vi "Logger.vi"(0 "Folder":path, 5 "Name":string, 7 "Level":T1=enum."Info", 9 "Retain (days)":i32=14, 11 "Length":i32=10000) -> ()   [LabVIEW 2020]
uses:
  Typedefs/Logger-Level.ctl
  Typedefs/Logger-Queue Data.ctl
  Typedefs/Logger-Action.ctl
  Typedefs/Logger-State.ctl
  Typedefs/Logger-Globals.vi
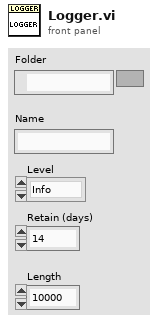
[diagram p1: front panel]
types:
  T1 = typedef "Logger-Level.ctl" = enum16{"Debug", "TCP", "Info", "Warning", "Error", "Critical"}
  T2 = typedef "Logger-Queue Data.ctl" = cluster{"Action":T3, "Level":T1, "Time":dbl, "Message":string}
  T3 = typedef "Logger-Action.ctl" = enum16{"None", "Init", "Add", "Show", "Offset", "Quit"}
  T4 = typedef "Logger-State.ctl" = cluster{"path":path, "index":i32, "log":u8[], "Offset (s)":dbl}
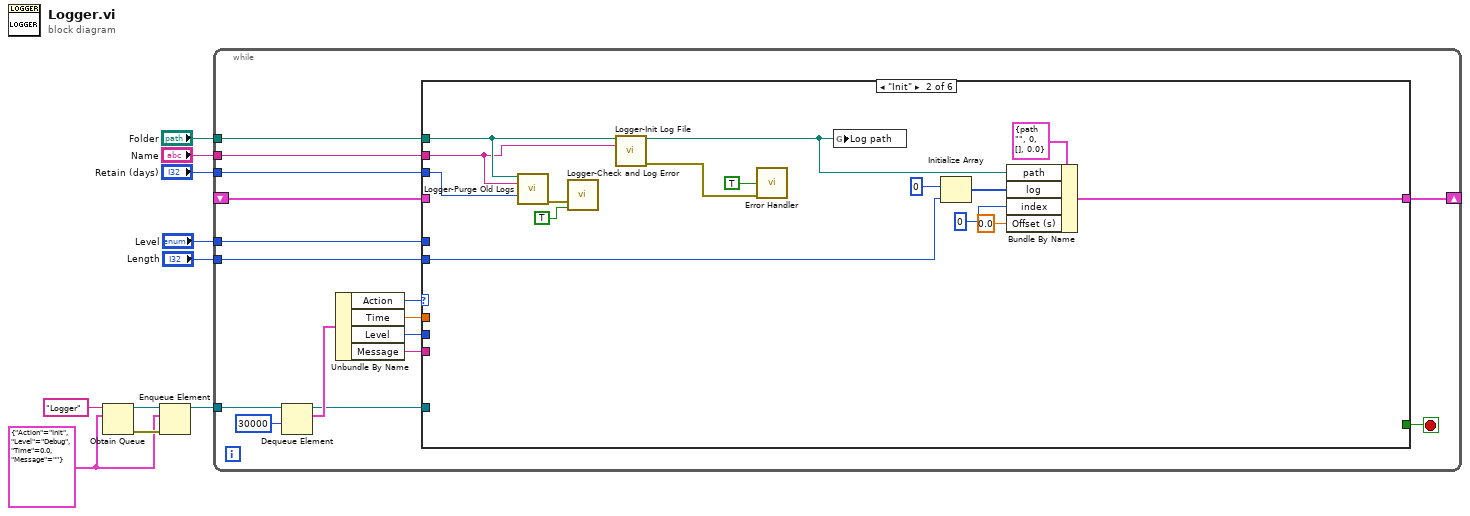
[diagram p0: block diagram]
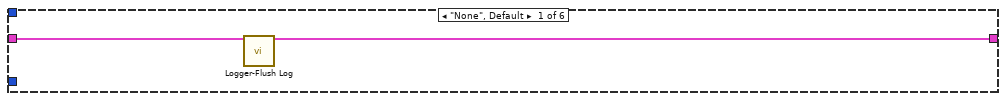
[diagram p2: hidden frame]
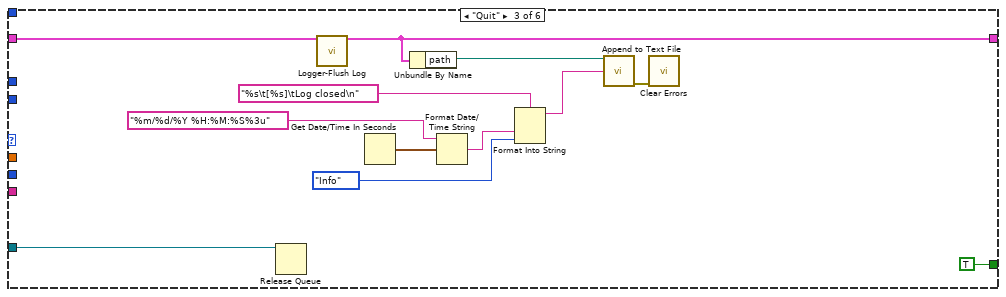
[diagram p3: hidden frame]
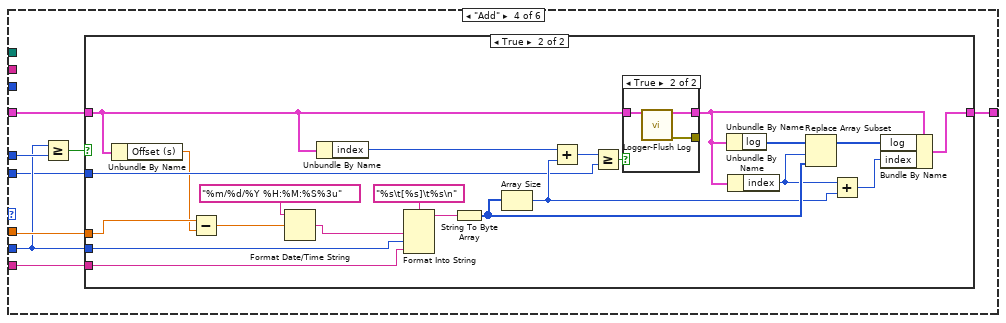
[diagram p4: hidden frame]
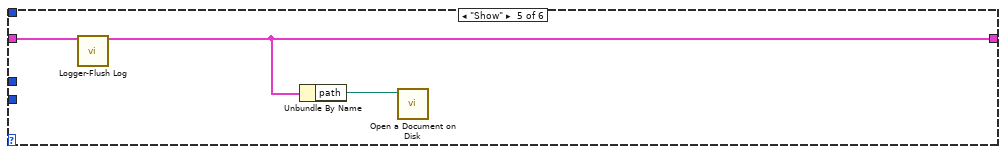
[diagram p7: hidden frame]
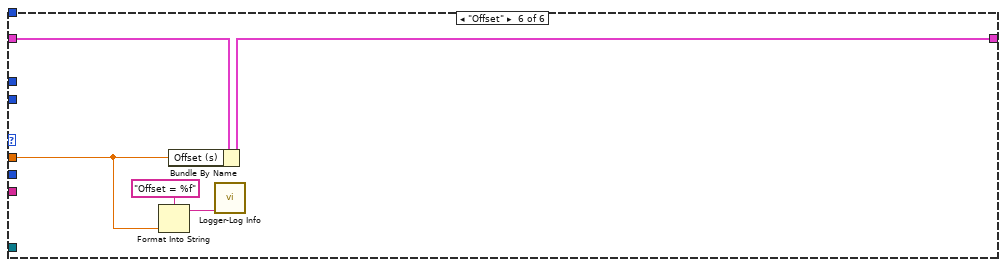
[diagram p8: hidden frame]
diagram:
  w4 = T2 {"Action"=enum."Init", "Level"=enum."Debug", "Time"=0.0, "Message"=""} ("Trace Data")
  n1 = Obtain Queue(name (unnamed)="Logger", element data type=w4) -> (queue out=w6:refnum<queue>, error out=w5:errorcluster)  [unwired: 3 in, 1 out]
  n2 = Enqueue Element(queue=w6, element=w4, error in (no error)=w5) -> (queue out=w7:refnum<queue>)  [unwired: 1 in, 2 out]
  n3 = while {
    tunnel: w7 -> [w26]
    shift-right: [w20] -> _
    shift-left: _ -> [w17]
    tunnel: "Level" -> [w16]
    tunnel: "Length" -> [w15]
    tunnel: "Name" -> [w14]
    tunnel: "Folder" -> [w13]
    tunnel: "Retain (days)" -> [w12]
    stop <- w21 stop-if-true
    n4 = Dequeue Element(queue=w26, timeout in ms (-1)=30000) -> (queue out=w22:refnum<queue>, element=w25:T2)  [unwired: 1 in, 2 out]
    n5 = Unbundle By Name(w25) -> ("Action"=w24:T3, "Time"=w23:dbl, "Level"=w18:T1, "Message"=w19:string)
    n6 = case shown="\"Init\"" w24 {
      tunnel: [_ _ TRUE _ _ _] -> w21
      tunnel: w23 -> [_ _ _ w63 _ w95]
      tunnel: w17 -> [w28 _ w53 w62 w92 w98]
      tunnel: w22 -> [_ _ w55 _ _ _]
      tunnel: [w27 w40 w47 w61 w91 w97] -> w20
      tunnel: w19 -> [_ _ _ w60 _ _]
      tunnel: w18 -> [_ _ _ w57 _ _]
      tunnel: w16 -> [_ _ _ w58 _ _]
      tunnel: w15 -> [_ w39 _ w56 _ _]
      tunnel: w14 -> [_ w34 _ _ _ _]
      tunnel: w13 -> [_ w35 _ _ _ _]
      tunnel: w12 -> [_ w37 _ _ _ _]
      frame "None", Default {
        n7 = call "Logger-Flush Log.vi"("State in"=w28) -> ("State out"=w27:T4)  [unwired: 13 in, 1 out]
      }
      frame "Init" {
        n8 = call "Logger-Purge Old Logs.vi"("Folder"=w35, "Name"=w34, "Retain (days)"=w37) -> ("error out"=w30:errorcluster)  [unwired: 12 in]
        n9 = call "Logger-Check and Log Error.vi"("error in (no error)"=w30, "Clear?"=TRUE) -> ()  [unwired: 13 in, 1 out]
        n10 = call "Logger-Init Log File.vi"("Folder"=w35, "Name"=w34) -> ("File path"=w32:path, "error out"=w36:errorcluster)  [unwired: 12 in]
        n11 = call "Error Handler.vi"("Log?"=TRUE, "error in (no error)"=w36) -> ()  [unwired: 11 in, 3 out]
        n12 = global write "Logger-Globals.vi" "Log path"(w32) -> ()
        n13 = Initialize Array(u8 0, w39) -> (w43:u8[])
        n14 = Bundle By Name(cluster=T4 {"path"=path "", "index"=0, "log"=[], "Offset (s)"=0.0} ("State"), "path"=w32, "log"=w43, "index"=0, "Offset (s)"=0.0) -> (w40:T4)
      }
      frame "Quit" {
        n15 = Release Queue(queue=w55) -> ()  [unwired: 2 in, 3 out]
        n16 = call "Logger-Flush Log.vi"("State in"=w53) -> ("State out"=w47:T4)  [unwired: 13 in, 1 out]
        n17 = Get Date/Time In Seconds() -> (seconds since 1Jan1904=w51:timestamp)
        n18 = Unbundle By Name(w47) -> ("path"=w46:path)
        n19 = Format Date/Time String(time format string (%c)="%m/%d/%Y %H:%M:%S%3u", seconds (now)=w51) -> (date/time string=w49:string)  [unwired: 1 in]
        n20 = Format Into String(format string="%s\t[%s]\tLog closed\n", w49, Logger-Level."Info" ("Level")) -> (resulting string=w45:string)  [unwired: 2 in, 1 out]
        n21 = call "Append to Text File.vi"("file path"=w46, "text"=w45) -> ("error out"=w44:errorcluster)  [unwired: 12 in, 1 out]
        n22 = call <vilib>:"Clear Errors.vi"("error in (no error)"=w44) -> ()  [unwired: 5 in, 2 out]
      }
      frame "Add" {
        n23 = Greater Or Equal?(x=w57, y=w58) -> (x >= y?=w59:bool)
        n24 = case shown="True" w59 {
          tunnel: w63 -> [_ w67]
          tunnel: w62 -> [w64 w66]
          tunnel: [w64 w83] -> w61
          tunnel: w60 -> [_ w73]
          tunnel: w57 -> [_ w72]
          tunnel: w56 -> [_ w71]
          frame False {
          }
          frame True {
            n25 = Unbundle By Name(w66) -> ("Offset (s)"=w65:dbl)
            n26 = Subtract(x=w67, y=w65) -> (x-y=w68:dbl)
            n27 = Format Date/Time String(time format string (%c)="%m/%d/%Y %H:%M:%S%3u", seconds (now)=w68) -> (date/time string=w69:string)  [unwired: 1 in]
            n28 = Unbundle By Name(w66) -> ("index"=w84:i32)
            n29 = Format Into String(format string="%s\t[%s]\t%s\n", w69, w72, w73) -> (resulting string=w85:string)  [unwired: 2 in, 1 out]
            n30 = String To Byte Array(string=w85) -> (unsigned byte array=w79:u8[])
            n31 = Array Size(array=w79) -> (size(s)=w74:i32)
            n32 = Add(x=w84, y=w74) -> (x+y=w82:i32)
            n33 = Greater Or Equal?(x=w82, y=w71) -> (x >= y?=w81:bool)
            n34 = case shown="True" w81 {
              tunnel: w66 -> [w87 w90]
              tunnel: [w87 w89] -> w77
              tunnel: [_ w88] -> _
              frame False {
              }
              frame True {
                n35 = call "Logger-Flush Log.vi"("State in"=w90) -> ("State out"=w89:T4, "error out"=w88:errorcluster)  [unwired: 13 in]
              }
            }
            n36 = Unbundle By Name(w77) -> ("log"=w80:u8[])
            n37 = Unbundle By Name(w77) -> ("index"=w76:i32)
            n38 = Replace Array Subset(array=w80, new element=w79, index=w76) -> (w78:u8[])
            n39 = Add(x=w76, y=w74) -> (x+y=w75:i32)
            n40 = Bundle By Name(cluster=w77, "log"=w78, "index"=w75) -> (w83:T4)
          }
        }
      }
      frame "Show" {
        n41 = call "Logger-Flush Log.vi"("State in"=w92) -> ("State out"=w91:T4)  [unwired: 13 in, 1 out]
        n42 = Unbundle By Name(w91) -> ("path"=w93:path)
        n43 = call <vilib>:"Open a Document on Disk.vi"("document path"=w93) -> ()  [unwired: 6 in, 1 out]
      }
      frame "Offset" {
        n44 = Format Into String(format string="Offset = %f", w95) -> (resulting string=w94:string)  [unwired: 2 in, 1 out]
        n45 = Bundle By Name(cluster=w98, "Offset (s)"=w95) -> (w97:T4)
        n46 = call "Logger-Log Info.vi"("Message"=w94) -> ()  [unwired: 14 in, 1 out]
      }
    }
  }
